vi "Create Request-JSONtext.vi"(6 "notification?":bool, 8 "error in (no error)":errorcluster, 9 "params":variant, 10 "method":string) -> (0 "error out":errorcluster, 2 "{JSON}":string, 4 "id":string)   [LabVIEW 2019, in "JSON-RPC.lvclass"]
uses:
  JSON-RPC.lvclass
  6cd1d572-2af6-48e8-9b38-c51782860e23.vi
  7c5521bf-cb07-444f-843e-f9f289aa2aae.vi
  f6ae5555-b15c-4e52-b9b9-d6341c380ca9.vi
  6eedbf92-275d-42c0-90bb-b913601e88e9.vi
  <vilib>/JDP Science/JSONtext/Variant to JSON Text.vi
  <vilib>/Utility/MD5Checksum.llb/MD5Checksum string.vi
  <vilib>/JDP Science/JSONtext/LVClass Serializer/JSONtext LVClass Serializer.lvclass
  <vilib>/Utility/Data Type/NI_Data Type.lvlib
  <vilib>/JDP Science/JSONtext/JSONtext.lvlib
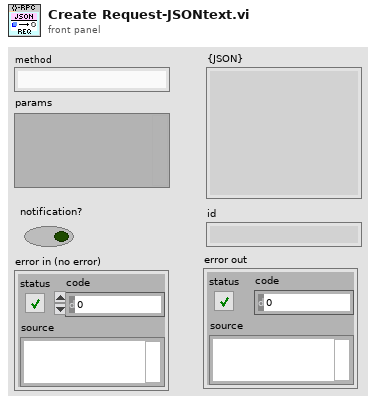
[diagram p1: front panel]
types:
  T1 = typedef "NI_Data Type.lvlib/Data Type.ctl" = enum8{"Invalid Type", "Void", "I8", "I16", "I32", "I64", "U8", "U16", "U32", "U64", "Single Float", "Double Float", "Extended Float", "Single Complex", "Double Complex", "Extended Complex", "Enum U8", "Enum U16", "Enum U32", "Enum U64", "Single Float With Unit", "Double Float With Unit", "Extended Float With Unit", "Single Complex with Unit", "Double Complex with Unit", "Extended Complex with Unit", "Boolean", "String", "Path", "Picture", "Tag", "Array", "Cluster", "Variant", "LV Variant", "Waveform", "Timestamp", "Digital Waveform", "Digital Data", "ExpressData", "Refnum", "External Data", "VI", "Poly VI", "LabVIEW Class Instance", "Fixed Point", "Set Collection", "Map Collection"}
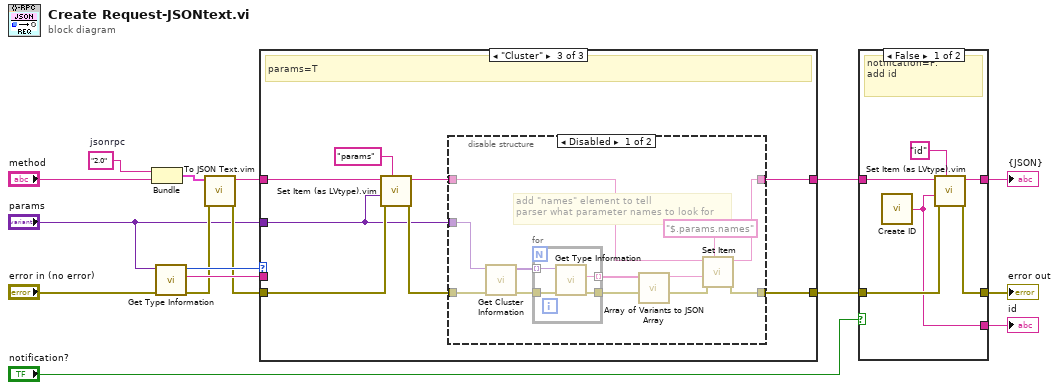
[diagram p0: block diagram]
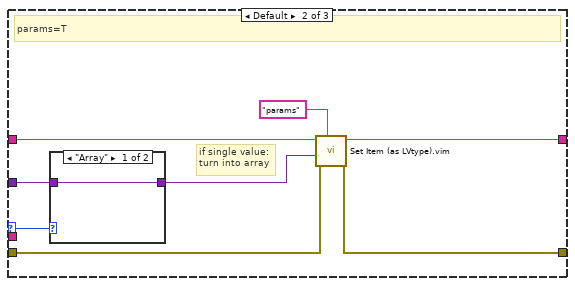
[diagram p3: hidden frame]
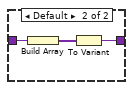
[diagram p4: hidden frame]
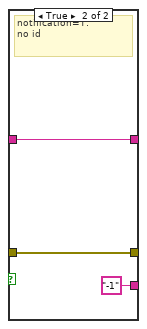
[diagram p6: hidden frame]
diagram:
  w6 = "2.0"  # jsonrpc
  n1 = Bundle("jsonrpc"=w6, "method"="method") -> (w7:cluster{"jsonrpc":string, "method":string})  [unwired: 1 in]
  n2 = call <vilib>:"Get Type Information.vi"("error in (no error)"="error in (no error)", "variant"="params") -> ("error out"=w4:errorcluster, "name"=w8:string, "type"=w12:T1)  [unwired: 5 in, 2 out]
  n3 = call "To JSON Text.vim"("error in (no error)"=w4, "Anything"=w7) -> ("error out"=w3:errorcluster, "<JSON>"=w2:string)  [unwired: 8 in]
  n4 = case shown="\"Cluster\"" w12 {
    selector: w12 -> [_ w25 _]
    tunnel: [w18 w21 w38] -> w10
    tunnel: [w17 w20 w37] -> w11
    tunnel: w3 -> [w18 w19 w34]
    tunnel: w2 -> [w17 w26 w35]
    tunnel: "params" -> [_ w24 w31]
    tunnel: w8 -> [_ _ _]
    frame "Void" {
      # "no params"
    }
    frame Default {
      # "if single value:\nturn into array"
      # "params=T"
      n5 = case shown="\"Array\"" w25 {
        tunnel: w24 -> [w27 w30]
        tunnel: [w27 w29] -> w22
        frame "Array" {
        }
        frame Default {
          n6 = Build Array(w30) -> (w28:variant[])
          n7 = To Variant(anything=w28) -> (Variant=w29:variant)
        }
      }
      n8 = call "Set Item (as LVtype).vim"("$Path or Item Name"="params" ("Object (or Item) Path"), "error in (no error)"=w19, "Anything"=w22, "JSON"=w26) -> ("error out"=w21:errorcluster, "<JSON>"=w20:string)  [unwired: 4 in, 1 out]
    }
    frame "Cluster" {
      # "params=T"
      n9 = call "Set Item (as LVtype).vim"("$Path or Item Name"="params" ("Object (or Item) Path"), "error in (no error)"=w34, "Anything"=w31, "JSON"=w35) -> ("error out"=w33:errorcluster, "<JSON>"=w32:string)  [unwired: 4 in, 1 out]
      n10 = disable-structure shown="Disabled" {
        disable-tunnel: [w47 w55] -> w38
        disable-tunnel: w31 -> [w43 _]
        disable-tunnel: w33 -> [w42 w55]
        disable-tunnel: w32 -> [w41 w56]
        disable-tunnel: [w39 w56] -> w37
        frame Disabled {
          # "add \"names\" element to tell\nparser what parameter names to look for"
          n11 = call <vilib>:"Get Cluster Information.vi"("error in (no error)"=w42, "variant"=w43) -> ("error out"=w50:errorcluster, "cluster elements"=w49:variant[])  [unwired: 8 in]
          n12 = for {
            tunnel: w49 -> [w54] mode=indexing
            tunnel: [w53] -> w44 mode=indexing
            tunnel: w50 -> [w52]
            tunnel: [w51] -> w40
            n13 = call <vilib>:"Get Type Information.vi"("error in (no error)"=w52, "variant"=w54) -> ("error out"=w51:errorcluster, "name"=w53:string)  [unwired: 5 in, 3 out]
          }
          n14 = call <vilib>:"Array of Variants to JSON Array.vi"("error in (no error)"=w40, "Array of Variants"=w44) -> ("error out"=w45:errorcluster, "<JSON>"=w46:string)  [unwired: 8 in]
          n15 = call <vilib>:"Set Item.vi"("$Path or Item Name"="$.params.names", "error in (no error)"=w45, "JSON to Insert"=w46, "JSON"=w41) -> ("error out"=w47:errorcluster, "<JSON>"=w39:string)  [unwired: 4 in, 1 out]
        }
        frame Enabled {
        }
      }
    }
  }
  n16 = case shown="False" "notification?" {
    tunnel: w11 -> [w62 w65]
    tunnel: [w61 w65] -> w15
    tunnel: w10 -> [w59 w64]
    tunnel: [w60 w64] -> w14
    tunnel: [w57 "-1" ("id")] -> w9
    frame False {
      # "notification=F:\nadd id"
      n17 = call "Create ID.vi"() -> ("id"=w57:string)
      n18 = call "Set Item (as LVtype).vim"("$Path or Item Name"="id", "error in (no error)"=w59, "Anything"=w57, "JSON"=w62) -> ("error out"=w60:errorcluster, "<JSON>"=w61:string)  [unwired: 4 in, 1 out]
    }
    frame True {
      # "notification=T:\nno id"
    }
  }
  "error out" <- w14
  "{JSON}" <- w15
  "id" <- w9
